vi "Searching_for_Locally_Optimal_Elongation-1.vi"(7 "[IN] Still connected\ntracks in group":T1, 8 "[IN] # of Track with\nSuch Problem Point":i32, 11 "[IN] Index of Previous Point\n(There the search stoped)":i32) -> (0 "[OUT] # of Track with\nOptimal Elongation":i32, 3 "[OUT] Index indside track \nof Optimal Elongation":i32)   [LabVIEW 2013]
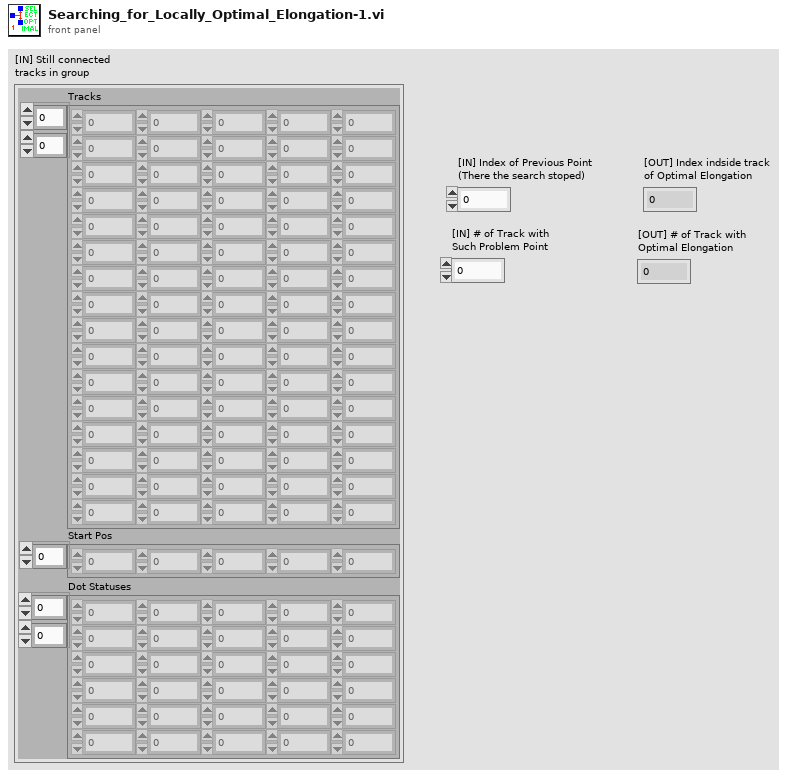
[diagram p1: front panel]
types:
  T1 = cluster{"Tracks":dbl[][], "Start Pos":i32[], "Dot Statuses":i16[][]}
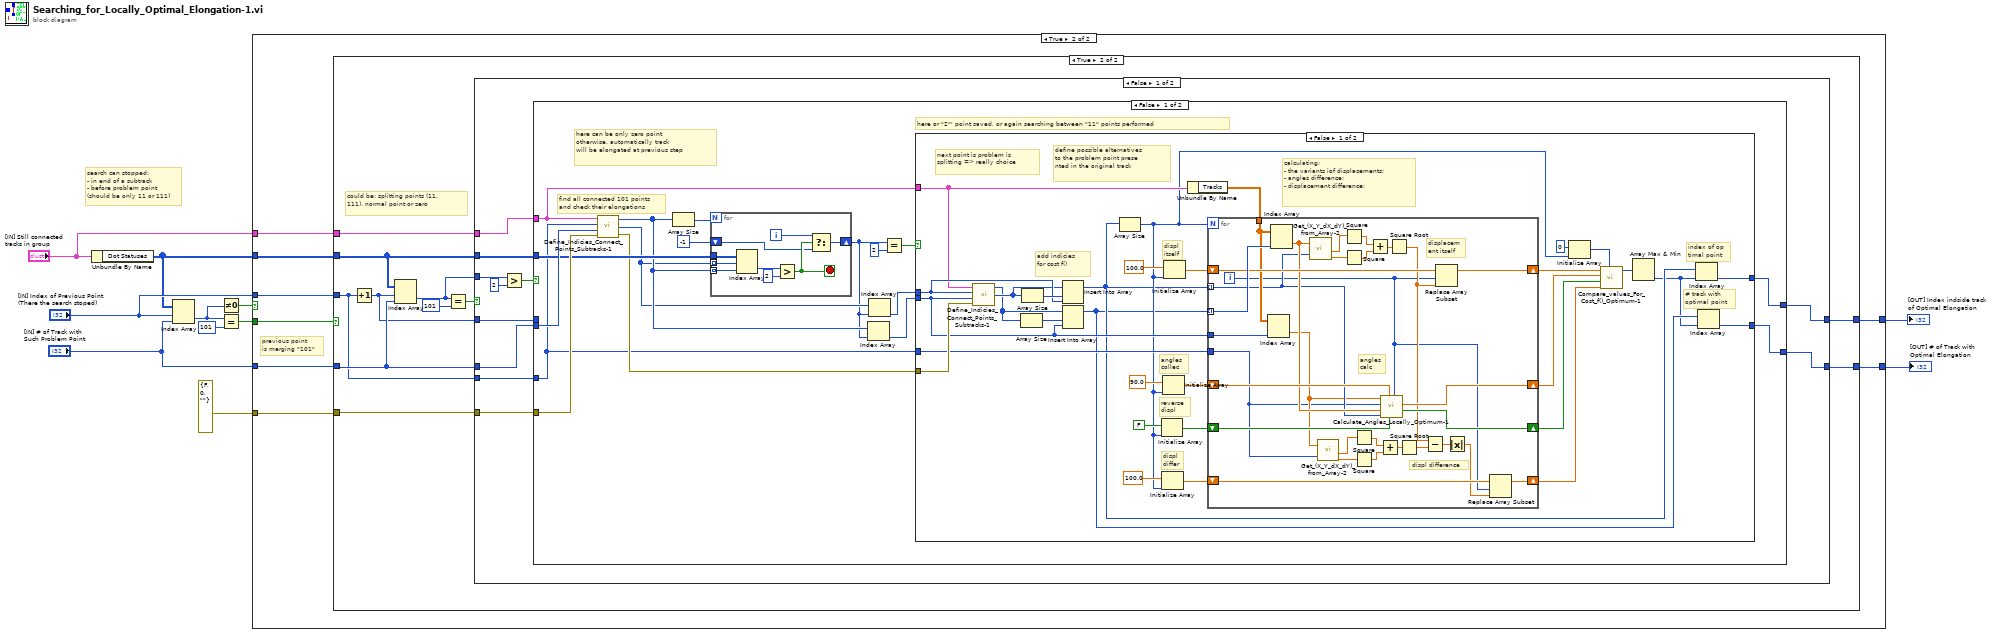
[diagram p0: block diagram]
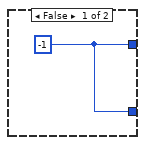
[diagram p2: hidden frame]
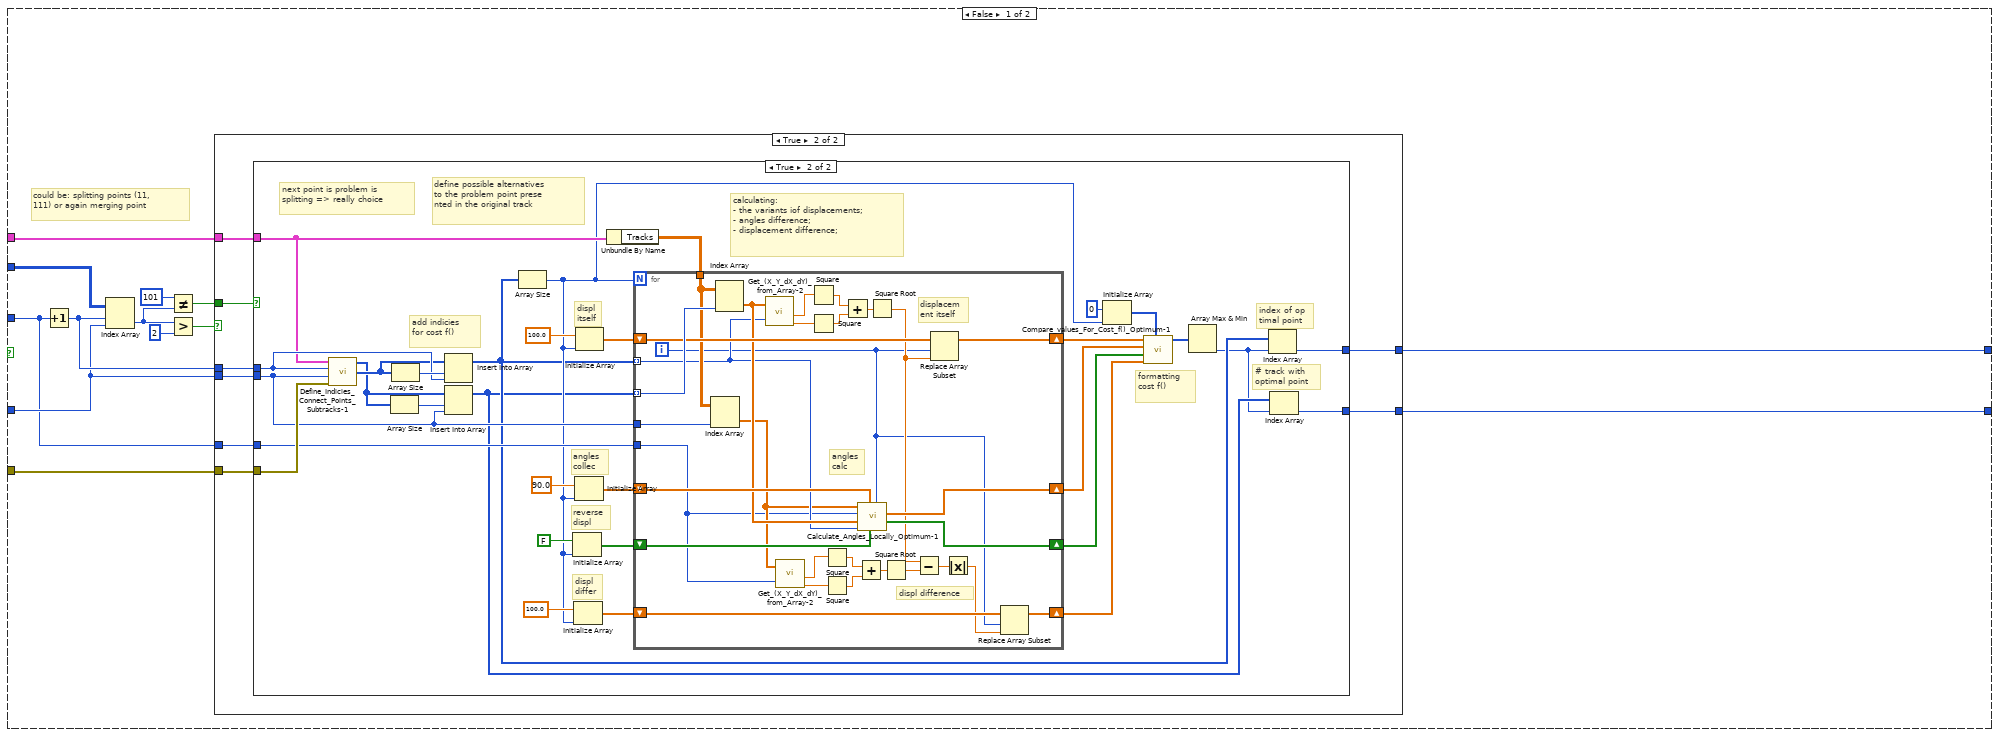
[diagram p3: hidden frame]
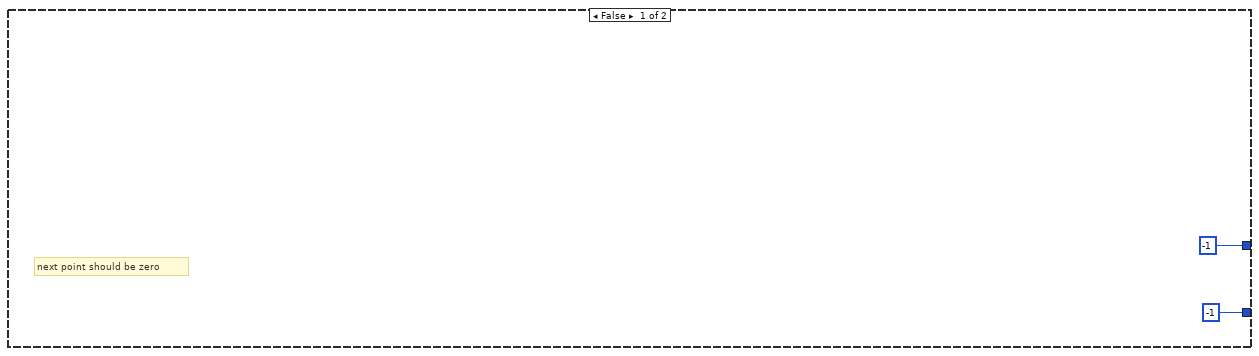
[diagram p4: hidden frame]
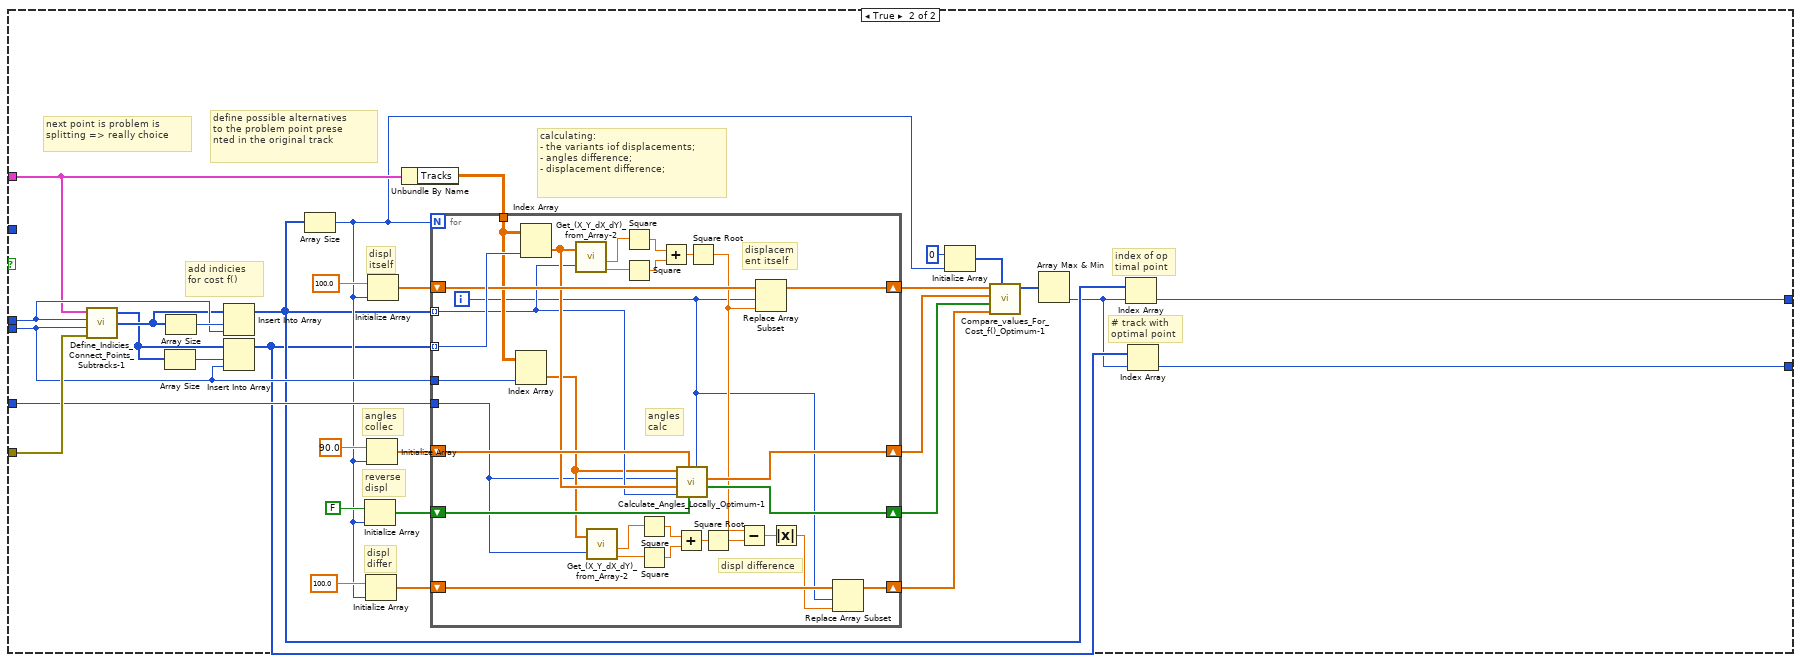
[diagram p7: hidden frame]
diagram:
  # "search can stopped: \n- in end of a subtrack\n- before problem point \n(should be only 11 or 111)"
  n1 = Unbundle By Name("[IN] Still connected\ntracks in group") -> ("Dot Statuses"=w8:i16[][])
  n2 = Index Array(array=w8, index (row)="[IN] Index of Previous Point\n(There the search stoped)", index (col)="[IN] # of Track with\nSuch Problem Point") -> (element=w2:i16)
  n3 = Not Equal To 0?(x=w2) -> (x != 0?=w1:bool)
  n4 = Equal?(x=w2, y=i16 101) -> (x = y?=w10:bool)
  n5 = case shown="True" w1 {
    tunnel: w10 -> [_ w20]
    tunnel: "[IN] Index of Previous Point\n(There the search stoped)" -> [_ w19]
    tunnel: w8 -> [_ w18]
    tunnel: "[IN] # of Track with\nSuch Problem Point" -> [_ w17]
    tunnel: "[IN] Still connected\ntracks in group" -> [_ w16]
    tunnel: errorcluster {"status"=FALSE, "code"=0, "source"=""} ("error IN") -> [_ w15]
    tunnel: [w12 w14] -> w4
    tunnel: [w12 w13] -> w3
    frame False {
      w12 = -1 ("disabled index (row)")
    }
    frame True {
      # "previous point \nis merging \"101\""
      n6 = case shown="True" w20 {
        tunnel: w19 -> [w23 w108]
        tunnel: w18 -> [w33 w107]
        tunnel: w17 -> [w25 w115]
        tunnel: w16 -> [w27 w109]
        tunnel: w15 -> [w24 w110]
        tunnel: [w22 w113] -> w14
        tunnel: [w21 w112] -> w13
        frame False {
          # "could be: splitting points (11,\n111) or again merging point"
          n7 = Increment(x=w23) -> (x+1=w26:i32)
          n8 = Index Array(array=w33, index (row)=w26, index (col)=w25) -> (element=w30:i16)
          n9 = Not Equal?(x=i16 101, y=w30) -> (x != y?=w28:bool)
          n10 = Greater?(x=w30, y=i16 2) -> (0:w31:bool)
          n11 = case shown="True" w31 {
            tunnel: w28 -> [_ w43]
            tunnel: w27 -> [_ w42]
            tunnel: w26 -> [_ w41]
            tunnel: w25 -> [_ w40]
            tunnel: w24 -> [_ w39]
            tunnel: w23 -> [_ w38]
            tunnel: [-1 ("disabled index (row)") w37] -> w22
            tunnel: [-1 ("disabled index (row)") w36] -> w21
            frame False {
              # "next point should be zero"
            }
            frame True {
              n12 = case shown="True" w43 {
                tunnel: w42 -> [_ w64]
                tunnel: w41 -> [w45 w74]
                tunnel: w40 -> [w44 w61]
                tunnel: w39 -> [_ w76]
                tunnel: w38 -> [_ w62]
                tunnel: [w45 w47] -> w37
                tunnel: [w44 w46] -> w36
                frame False {
                  # "101 point itself serves as elongation"
                }
                frame True {
                  # "formatting\ncost f()"
                  # "# track with \noptimal point"
                  # "index of op\ntimal point"
                  # "displ\ndiffer"
                  # "calculating: \n- the variants iof displacements;\n- angles difference; \n- displacement difference;"
                  # "reverse \ndispl"
                  # "angles \ncollec"
                  # "displ\nitself"
                  # "add indicies \nfor cost f()"
                  # "define possible alternatives \nto the problem point prese\nnted in the original track"
                  # "next point is problem is \nsplitting => really choice"
                  n13 = call "Define_Indicies_Connect_Points_Subtracks-1.vi"("error IN"=w76, "[IN] Index of track with\n(problem displacement)"=w61, "[IN] Index of problem\ndisplacement inside track"=w74, "[IN] Track group"=w64) -> ("[OUT] Index of \nconnected dots\ninside the track"=w73:i32[], "[OUT] Index of connected\ntracks with problem dot"=w71:i32[])  [unwired: 1 out]
                  n14 = Array Size(array=w71) -> (size(s)=w72:i32)
                  n15 = Array Size(array=w73) -> (size(s)=w75:i32)
                  n16 = Insert Into Array(array=w73, index=w75, new element=w74) -> (w50:i32[])
                  n17 = Insert Into Array(array=w71, index=w72, new element=w61) -> (w49:i32[])
                  n18 = Array Size(array=w50) -> (size(s)=w57:i32)
                  n19 = Initialize Array(FALSE, w57) -> (w67:bool[])
                  n20 = Initialize Array(100.0 ("element"), w57) -> (w59:dbl[])
                  n21 = Initialize Array(90.0, w57) -> (w66:dbl[])
                  n22 = Initialize Array(100.0 ("element"), w57) -> (w65:dbl[])
                  n23 = Unbundle By Name(w64) -> ("Tracks"=w63:dbl[][])
                  n24 = for {
                    N: w57 -> [_]
                    shift-right: [w91] -> w53
                    shift-left: w67 -> [w96]
                    shift-right: [w92] -> w54
                    shift-left: w66 -> [w95]
                    shift-right: [w99] -> w56
                    shift-left: w65 -> [w100]
                    tunnel: w63 -> [w98]
                    tunnel: w50 -> [w93] mode=indexing
                    tunnel: w49 -> [w101] mode=indexing
                    tunnel: w62 -> [w84]
                    tunnel: w61 -> [w97]
                    shift-right: [w77] -> w52
                    shift-left: w59 -> [w80]
                    i -> [w78]
                    # "displacem\nent itself"
                    # "angles\ncalc"
                    # "displ difference"
                    n25 = Index Array(array=w98, index (col)=w97) -> (element=w87:dbl[])  [unwired: 1 in]
                    n26 = Index Array(array=w98, index (col)=w101) -> (element=w94:dbl[])  [unwired: 1 in]
                    n27 = call "Get_(X_Y_dX_dY)_from_Array-2.vi"("(X,Y,dX,dY)"=w94, "Index of Displacement"=w93) -> ("dX"=w104:dbl, "dY"=w103:dbl)  [unwired: 2 out]
                    n28 = call "Get_(X_Y_dX_dY)_from_Array-2.vi"("(X,Y,dX,dY)"=w87, "Index of Displacement"=w84) -> ("dX"=w88:dbl, "dY"=w86:dbl)  [unwired: 2 out]
                    n29 = Square(x=w104) -> (x^2=w106:dbl)
                    n30 = Square(x=w103) -> (x^2=w102:dbl)
                    n31 = Square(x=w88) -> (x^2=w90:dbl)
                    n32 = Square(x=w86) -> (x^2=w85:dbl)
                    n33 = Add(x=w106, y=w102) -> (x+y=w105:dbl)
                    n34 = Add(x=w90, y=w85) -> (x+y=w89:dbl)
                    n35 = call "Calculate_Angles_Locally_Optimum-1.vi"("[IN] Index of subtrack"=w78, "[IN] Reverse Displ or Not"=w96, "[IN] Array with Angles \nBetween Displacement"=w95, "[IN] Index of Cur\nrent Displacement"=w93, "[IN] Track with \nCurrent Point"=w94, "[IN] Index of Previ\nous Displacement"=w84, "[IN] Track with \nPrevious Point"=w87) -> ("[OUT] Reverse displacement or not"=w91:bool[], "[OUT] Angles betwe\nen two displacements"=w92:dbl[])  [unwired: 3 in]
                    n36 = Square Root(x=w105) -> (sqrt(x)=w82:dbl)
                    n37 = Square Root(x=w89) -> (sqrt(x)=w83:dbl)
                    n38 = Subtract(x=w82, y=w83) -> (x-y=w81:dbl)
                    n39 = Replace Array Subset(array=w100, new element=w82, index=w78) -> (w99:dbl[])
                    n40 = Absolute Value(x=w81) -> (abs(x)=w79:dbl)
                    n41 = Replace Array Subset(array=w80, new element=w79, index=w78) -> (w77:dbl[])
                  }
                  n42 = Initialize Array(i8 0 ("element"), w57) -> (w55:i8[])
                  n43 = call "Compare_values_For_Cost_f()_Optimum-1.vi"("[IN] Cost function"=w55, "[IN] Displ \ndifferences"=w52, "[IN] Reverse or not"=w53, "[IN] Angles betwe\nen displacements"=w54, "[IN] Array of displacements"=w56) -> ("[OUT] Cost function"=w51:i8[])  [unwired: 6 in]
                  n44 = Array Max & Min(array=w51) -> (min index (indices)=w48:i32)  [unwired: 3 out]
                  n45 = Index Array(array=w50, index=w48) -> (element=w47:i32)
                  n46 = Index Array(array=w49, index=w48) -> (element=w46:i32)
                }
              }
            }
          }
        }
        frame True {
          # "could be: splitting points (11,\n111), normal point or zero"
          n47 = Increment(x=w108) -> (x+1=w114:i32)
          n48 = Index Array(array=w107, index (row)=w114, index (col)=w115) -> (element=w111:i16)
          n49 = Equal?(x=w111, y=i16 101) -> (x = y?=w116:bool)
          n50 = case shown="False" w116 {
            tunnel: w115 -> [w124 w279]
            tunnel: w114 -> [w123 w280]
            tunnel: [w120 w280] -> w113
            tunnel: [w119 w279] -> w112
            tunnel: w111 -> [w127 _]
            tunnel: w110 -> [w125 _]
            tunnel: w109 -> [w122 _]
            tunnel: w108 -> [w121 _]
            tunnel: w107 -> [w118 _]
            frame False {
              n51 = Greater?(x=w127, y=i16 2) -> (0:w126:bool)
              n52 = case shown="False" w126 {
                tunnel: w122 -> [w138 w236]
                tunnel: w123 -> [_ w246]
                tunnel: w124 -> [w144 w233]
                tunnel: w125 -> [w145 w248]
                tunnel: w121 -> [w136 w234]
                tunnel: [w130 w219] -> w120
                tunnel: [w129 w218] -> w119
                tunnel: w118 -> [w142 _]
                frame False {
                  # "here or \"2\"' point saved, or again searching between \"11\" points performed"
                  # "here can be only zero point\notherwise, automatically track\nwill be elongated at previous step"
                  # "find all connected 101 points\nand check their elongations"
                  n53 = call "Define_Indicies_Connect_Points_Subtracks-1.vi"("error IN"=w145, "[IN] Index of track with\n(problem displacement)"=w144, "[IN] Index of problem\ndisplacement inside track"=w136, "[IN] Track group"=w138) -> ("error OUT"=w137:errorcluster, "[OUT] Index of \nconnected dots\ninside the track"=w134:i32[], "[OUT] Index of connected\ntracks with problem dot"=w135:i32[])
                  n54 = Array Size(array=w135) -> (size(s)=w143:i32)
                  n55 = for {
                    N: w143 -> [_]
                    tunnel: w135 -> [w216] mode=indexing
                    tunnel: w142 -> [w217]
                    tunnel: w134 -> [w215] mode=indexing
                    shift-right: [w209] -> w133
                    shift-left: -1 -> [w211]
                    i -> [w210]
                    stop <- w212 stop-if-true
                    n56 = Index Array(array=w217, index (row)=w215, index (col)=w216) -> (element=w214:i16)
                    n57 = Greater?(x=w214, y=i16 2) -> (0:w212:bool)
                    n58 = Select(t=w210, s=w212, f=w211) -> (s? t:f=w209:i32)
                  }
                  n59 = Index Array(array=w135, index=w133) -> (element=w131:i32)
                  n60 = Index Array(array=w134, index=w133) -> (element=w132:i32)
                  n61 = Equal?(x=w133, y=2) -> (x = y?=w139:bool)
                  n62 = case shown="False" w139 {
                    tunnel: w138 -> [w164 _]
                    tunnel: w132 -> [w174 w208]
                    tunnel: w131 -> [w161 w207]
                    tunnel: w137 -> [w176 _]
                    tunnel: w136 -> [w162 _]
                    tunnel: [w147 w208] -> w130
                    tunnel: [w146 w207] -> w129
                    frame False {
                      # "# track with \noptimal point"
                      # "index of op\ntimal point"
                      # "displ\ndiffer"
                      # "calculating: \n- the variants iof displacements;\n- angles difference; \n- displacement difference;"
                      # "reverse \ndispl"
                      # "angles \ncollec"
                      # "displ\nitself"
                      # "add indicies \nfor cost f()"
                      # "define possible alternatives \nto the problem point prese\nnted in the original track"
                      # "next point is problem is \nsplitting => really choice"
                      n63 = call "Define_Indicies_Connect_Points_Subtracks-1.vi"("error IN"=w176, "[IN] Index of track with\n(problem displacement)"=w161, "[IN] Index of problem\ndisplacement inside track"=w174, "[IN] Track group"=w164) -> ("[OUT] Index of \nconnected dots\ninside the track"=w173:i32[], "[OUT] Index of connected\ntracks with problem dot"=w171:i32[])  [unwired: 1 out]
                      n64 = Array Size(array=w171) -> (size(s)=w172:i32)
                      n65 = Array Size(array=w173) -> (size(s)=w175:i32)
                      n66 = Insert Into Array(array=w173, index=w175, new element=w174) -> (w150:i32[])
                      n67 = Insert Into Array(array=w171, index=w172, new element=w161) -> (w149:i32[])
                      n68 = Array Size(array=w150) -> (size(s)=w157:i32)
                      n69 = Initialize Array(FALSE, w157) -> (w167:bool[])
                      n70 = Initialize Array(100.0 ("element"), w157) -> (w159:dbl[])
                      n71 = Initialize Array(90.0, w157) -> (w166:dbl[])
                      n72 = Initialize Array(100.0 ("element"), w157) -> (w165:dbl[])
                      n73 = Unbundle By Name(w164) -> ("Tracks"=w163:dbl[][])
                      n74 = for {
                        N: w157 -> [_]
                        shift-right: [w191] -> w153
                        shift-left: w167 -> [w196]
                        shift-right: [w192] -> w154
                        shift-left: w166 -> [w195]
                        shift-right: [w199] -> w156
                        shift-left: w165 -> [w200]
                        tunnel: w163 -> [w198]
                        tunnel: w150 -> [w193] mode=indexing
                        tunnel: w149 -> [w201] mode=indexing
                        tunnel: w162 -> [w184]
                        tunnel: w161 -> [w197]
                        shift-right: [w177] -> w152
                        shift-left: w159 -> [w180]
                        i -> [w178]
                        # "displacem\nent itself"
                        # "angles\ncalc"
                        # "displ difference"
                        n75 = Index Array(array=w198, index (col)=w197) -> (element=w187:dbl[])  [unwired: 1 in]
                        n76 = Index Array(array=w198, index (col)=w201) -> (element=w194:dbl[])  [unwired: 1 in]
                        n77 = call "Get_(X_Y_dX_dY)_from_Array-2.vi"("(X,Y,dX,dY)"=w194, "Index of Displacement"=w193) -> ("dX"=w204:dbl, "dY"=w203:dbl)  [unwired: 2 out]
                        n78 = call "Get_(X_Y_dX_dY)_from_Array-2.vi"("(X,Y,dX,dY)"=w187, "Index of Displacement"=w184) -> ("dX"=w188:dbl, "dY"=w186:dbl)  [unwired: 2 out]
                        n79 = Square(x=w204) -> (x^2=w206:dbl)
                        n80 = Square(x=w203) -> (x^2=w202:dbl)
                        n81 = Square(x=w188) -> (x^2=w190:dbl)
                        n82 = Square(x=w186) -> (x^2=w185:dbl)
                        n83 = Add(x=w206, y=w202) -> (x+y=w205:dbl)
                        n84 = Add(x=w190, y=w185) -> (x+y=w189:dbl)
                        n85 = call "Calculate_Angles_Locally_Optimum-1.vi"("[IN] Index of subtrack"=w178, "[IN] Reverse Displ or Not"=w196, "[IN] Array with Angles \nBetween Displacement"=w195, "[IN] Index of Cur\nrent Displacement"=w193, "[IN] Track with \nCurrent Point"=w194, "[IN] Index of Previ\nous Displacement"=w184, "[IN] Track with \nPrevious Point"=w187) -> ("[OUT] Reverse displacement or not"=w191:bool[], "[OUT] Angles betwe\nen two displacements"=w192:dbl[])  [unwired: 3 in]
                        n86 = Square Root(x=w205) -> (sqrt(x)=w182:dbl)
                        n87 = Square Root(x=w189) -> (sqrt(x)=w183:dbl)
                        n88 = Subtract(x=w182, y=w183) -> (x-y=w181:dbl)
                        n89 = Replace Array Subset(array=w200, new element=w182, index=w178) -> (w199:dbl[])
                        n90 = Absolute Value(x=w181) -> (abs(x)=w179:dbl)
                        n91 = Replace Array Subset(array=w180, new element=w179, index=w178) -> (w177:dbl[])
                      }
                      n92 = Initialize Array(i8 0 ("element"), w157) -> (w155:i8[])
                      n93 = call "Compare_values_For_Cost_f()_Optimum-1.vi"("[IN] Cost function"=w155, "[IN] Displ \ndifferences"=w152, "[IN] Reverse or not"=w153, "[IN] Angles betwe\nen displacements"=w154, "[IN] Array of displacements"=w156) -> ("[OUT] Cost function"=w151:i8[])  [unwired: 6 in]
                      n94 = Array Max & Min(array=w151) -> (min index (indices)=w148:i32)  [unwired: 3 out]
                      n95 = Index Array(array=w150, index=w148) -> (element=w147:i32)
                      n96 = Index Array(array=w149, index=w148) -> (element=w146:i32)
                    }
                    frame True {
                      # "some \"2\" point found\nit can be used as elongation"
                    }
                  }
                }
                frame True {
                  # "# track with \noptimal point"
                  # "index of op\ntimal point"
                  # "displ\ndiffer"
                  # "calculating: \n- the variants iof displacements;\n- angles difference; \n- displacement difference;"
                  # "reverse \ndispl"
                  # "angles \ncollec"
                  # "displ\nitself"
                  # "add indicies \nfor cost f()"
                  # "define possible alternatives \nto the problem point prese\nnted in the original track"
                  # "next point is problem is \nsplitting => really choice"
                  n97 = call "Define_Indicies_Connect_Points_Subtracks-1.vi"("error IN"=w248, "[IN] Index of track with\n(problem displacement)"=w233, "[IN] Index of problem\ndisplacement inside track"=w246, "[IN] Track group"=w236) -> ("[OUT] Index of \nconnected dots\ninside the track"=w245:i32[], "[OUT] Index of connected\ntracks with problem dot"=w243:i32[])  [unwired: 1 out]
                  n98 = Array Size(array=w243) -> (size(s)=w244:i32)
                  n99 = Array Size(array=w245) -> (size(s)=w247:i32)
                  n100 = Insert Into Array(array=w245, index=w247, new element=w246) -> (w222:i32[])
                  n101 = Insert Into Array(array=w243, index=w244, new element=w233) -> (w221:i32[])
                  n102 = Array Size(array=w222) -> (size(s)=w229:i32)
                  n103 = Initialize Array(FALSE, w229) -> (w239:bool[])
                  n104 = Initialize Array(100.0 ("element"), w229) -> (w231:dbl[])
                  n105 = Initialize Array(90.0, w229) -> (w238:dbl[])
                  n106 = Initialize Array(100.0 ("element"), w229) -> (w237:dbl[])
                  n107 = Unbundle By Name(w236) -> ("Tracks"=w235:dbl[][])
                  n108 = for {
                    N: w229 -> [_]
                    shift-right: [w263] -> w225
                    shift-left: w239 -> [w268]
                    shift-right: [w264] -> w226
                    shift-left: w238 -> [w267]
                    shift-right: [w271] -> w228
                    shift-left: w237 -> [w272]
                    tunnel: w235 -> [w270]
                    tunnel: w222 -> [w265] mode=indexing
                    tunnel: w221 -> [w273] mode=indexing
                    tunnel: w234 -> [w256]
                    tunnel: w233 -> [w269]
                    shift-right: [w249] -> w224
                    shift-left: w231 -> [w252]
                    i -> [w250]
                    # "displacem\nent itself"
                    # "angles\ncalc"
                    # "displ difference"
                    n109 = Index Array(array=w270, index (col)=w269) -> (element=w259:dbl[])  [unwired: 1 in]
                    n110 = Index Array(array=w270, index (col)=w273) -> (element=w266:dbl[])  [unwired: 1 in]
                    n111 = call "Get_(X_Y_dX_dY)_from_Array-2.vi"("(X,Y,dX,dY)"=w266, "Index of Displacement"=w265) -> ("dX"=w276:dbl, "dY"=w275:dbl)  [unwired: 2 out]
                    n112 = call "Get_(X_Y_dX_dY)_from_Array-2.vi"("(X,Y,dX,dY)"=w259, "Index of Displacement"=w256) -> ("dX"=w260:dbl, "dY"=w258:dbl)  [unwired: 2 out]
                    n113 = Square(x=w276) -> (x^2=w278:dbl)
                    n114 = Square(x=w275) -> (x^2=w274:dbl)
                    n115 = Square(x=w260) -> (x^2=w262:dbl)
                    n116 = Square(x=w258) -> (x^2=w257:dbl)
                    n117 = Add(x=w278, y=w274) -> (x+y=w277:dbl)
                    n118 = Add(x=w262, y=w257) -> (x+y=w261:dbl)
                    n119 = call "Calculate_Angles_Locally_Optimum-1.vi"("[IN] Index of subtrack"=w250, "[IN] Reverse Displ or Not"=w268, "[IN] Array with Angles \nBetween Displacement"=w267, "[IN] Index of Cur\nrent Displacement"=w265, "[IN] Track with \nCurrent Point"=w266, "[IN] Index of Previ\nous Displacement"=w256, "[IN] Track with \nPrevious Point"=w259) -> ("[OUT] Reverse displacement or not"=w263:bool[], "[OUT] Angles betwe\nen two displacements"=w264:dbl[])  [unwired: 3 in]
                    n120 = Square Root(x=w277) -> (sqrt(x)=w254:dbl)
                    n121 = Square Root(x=w261) -> (sqrt(x)=w255:dbl)
                    n122 = Subtract(x=w254, y=w255) -> (x-y=w253:dbl)
                    n123 = Replace Array Subset(array=w272, new element=w254, index=w250) -> (w271:dbl[])
                    n124 = Absolute Value(x=w253) -> (abs(x)=w251:dbl)
                    n125 = Replace Array Subset(array=w252, new element=w251, index=w250) -> (w249:dbl[])
                  }
                  n126 = Initialize Array(i8 0 ("element"), w229) -> (w227:i8[])
                  n127 = call "Compare_values_For_Cost_f()_Optimum-1.vi"("[IN] Cost function"=w227, "[IN] Displ \ndifferences"=w224, "[IN] Reverse or not"=w225, "[IN] Angles betwe\nen displacements"=w226, "[IN] Array of displacements"=w228) -> ("[OUT] Cost function"=w223:i8[])  [unwired: 6 in]
                  n128 = Array Max & Min(array=w223) -> (min index (indices)=w220:i32)  [unwired: 3 out]
                  n129 = Index Array(array=w222, index=w220) -> (element=w219:i32)
                  n130 = Index Array(array=w221, index=w220) -> (element=w218:i32)
                }
              }
            }
            frame True {
              # "\"101\"point serves as elongation"
            }
          }
        }
      }
    }
  }
  "[OUT] Index indside track \nof Optimal Elongation" <- w4
  "[OUT] # of Track with\nOptimal Elongation" <- w3
